vi "read_spectrum_txt_file.vi"(11 "File path":path) -> (1 "Spectrum Graph":cluster{"Y":dbl[], "Y":dbl[]}[](graph), 3 "File Name":path)   [LabVIEW 2009]
uses:
  <vilib>/Utility/file.llb/Read From Spreadsheet File (DBL).vi
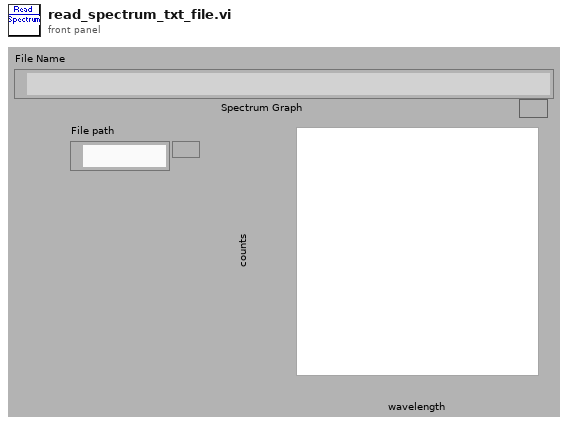
[diagram p1: front panel]
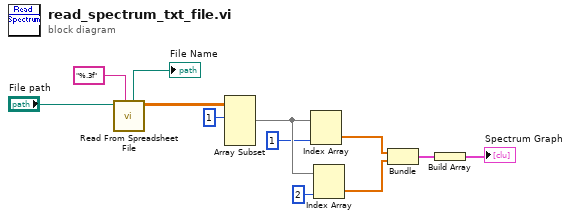
[diagram p0: block diagram]
diagram:
  n1 = call-poly <vilib>:"Read From Spreadsheet File.vi"("format (%.3f)"="%.3f", "file path (dialog if empty)"="File path") -> ("all rows"=w3:dbl[][], "new file path (Not A Path if cancelled)"=→"File Name":path)  [unwired: 5 in, 3 out]
  n2 = Array Subset(array=w3, index (row)=1) -> (w8:dbl[][])  [unwired: 3 in]
  n3 = Index Array(array=w8, index (col)=1 ("index (row)")) -> (element=w7:dbl[])  [unwired: 1 in]
  n4 = Index Array(array=w8, index (col)=2 ("disabled index (col)")) -> (element=w6:dbl[])  [unwired: 1 in]
  n5 = Bundle(w7, w6) -> (w5:cluster{dbl[], dbl[]})  [unwired: 1 in]
  n6 = Build Array(w5) -> (→"Spectrum Graph":cluster{dbl[], dbl[]}[])
